vi "panel.vi"(11 "面板属性":T1(array[cluster]) {"panle"."ID" min=1}) -> ()   [LabVIEW 2019]
panel:
  # "面板"
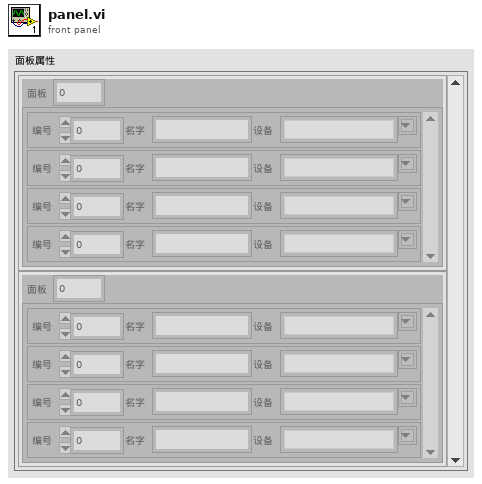
[diagram p1: front panel]
types:
  T1 = cluster{"id":dbl, "panle":cluster{"ID":u8, "Name":string, "Attribute":string}[]}[]
  T2 = cluster{"ID":u8, "Name":string, "Attribute":string}[]
  T3 = cluster{"id":dbl, "panle":cluster{"ID":u8, "Name":string, "Attribute":string}[]}
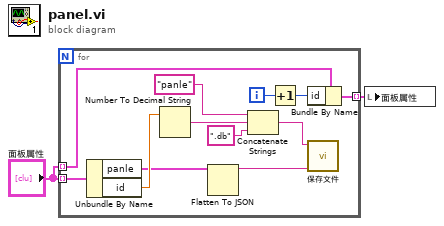
[diagram p0: block diagram]
diagram:
  n1 = for {
    tunnel: "面板属性" -> [w14] mode=indexing
    tunnel: [w13] -> w2 mode=indexing
    tunnel: "面板属性" -> [w10] mode=indexing
    i -> [w11]
    n2 = Unbundle By Name(w10) -> ("panle"=w5:T2, "id"=w9:dbl)
    n3 = Number To Decimal String(number=w9) -> (decimal integer string=w8:string)  [unwired: 1 in]
    n4 = Flatten To JSON(anything=w5) -> (JSON string=w4:string)  [unwired: 2 in, 1 out]
    n5 = Concatenate Strings("panle", w8, ".db") -> (w3:string)
    n6 = Increment(x=w11) -> (x+1=w12:i32)
    n7 = Bundle By Name(cluster=w14, "id"=w12) -> (w13:T3)
    n8 = call "保存文件.vi"("input"=w4, "文件名"=w3) -> ()  [unwired: 9 in, 1 out]
  }
  n9 = local write "面板属性"(w2) -> ()
